vi "Data Filter.vi"(9 "ZeroOffset":i32, 11 "Data":T1[](array[typedef]) {"Direction" items=["Tx", "Rx"]; "CANType" items=["CAN", "CANFD", "CANFD加速"]}) -> (1 "ZeroOffset out":i32, 3 "Data out":T1[](array[typedef]) {"Direction" items=["Tx", "Rx"]; "CANType" items=["CAN", "CANFD", "CANFD加速"]})   [LabVIEW 2018, in "CAN FD.lvlib"]
uses:
  CAN FD.lvlib
  Typedef/CAN Data.ctl
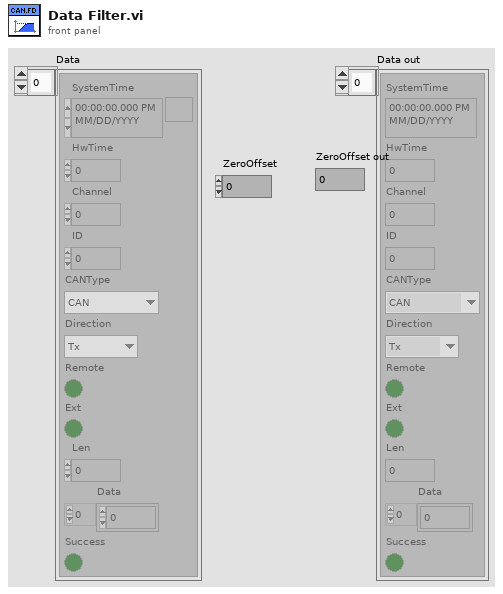
[diagram p1: front panel]
types:
  T1 = typedef "CAN FD.lvlib/CAN Data.ctl" = cluster{"SystemTime":timestamp, "HwTime":dbl, "Channel":u8, "ID":u32, "CANType":i16, "Direction":i16, "Remote":bool, "Ext":bool, "Len":u8, "Data":u8[], "Success":bool}
  T2 = cluster{"Channel":u8, "CANType":i16, "ID":u32, "Direction":i16}[]
  T3 = typedef "CAN FD.lvlib/Config.ctl" = cluster{"TimeFormat":u16, "ID Format":u16, "Data Format":u16, "ListLen":u32}
  T4 = typedef "CAN FD.lvlib/ListFilter.ctl" = cluster{"Timestamp":string, "Channel":string, "ID":string, "Type":i16, "Format":i16, "CANType":i16, "Direction":i16, "Len":string, "Data":string}
  T5 = cluster{"Channel":u8, "CANType":i16, "ID":u32, "Direction":i16}
  T6 = cluster{cluster{"Channel":u8, "CANType":i16, "ID":u32, "Direction":i16}, i32}
  T7 = cluster{cluster{"Channel":u8, "CANType":i16, "ID":u32, "Direction":i16}, i32}[]
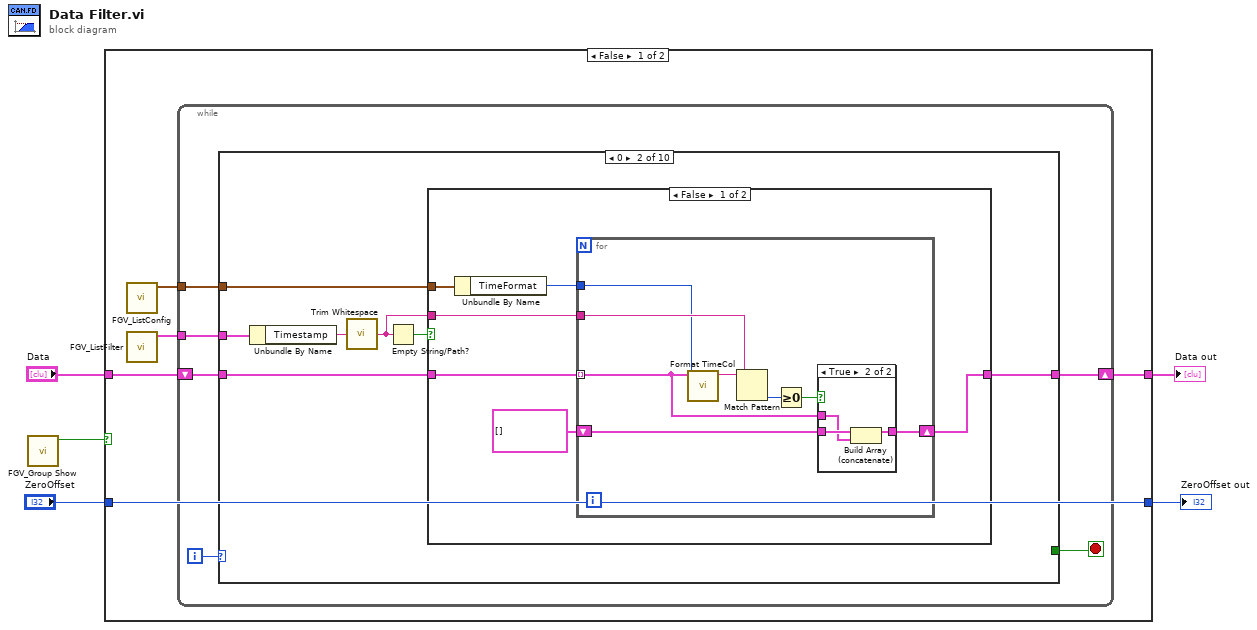
[diagram p0: block diagram]
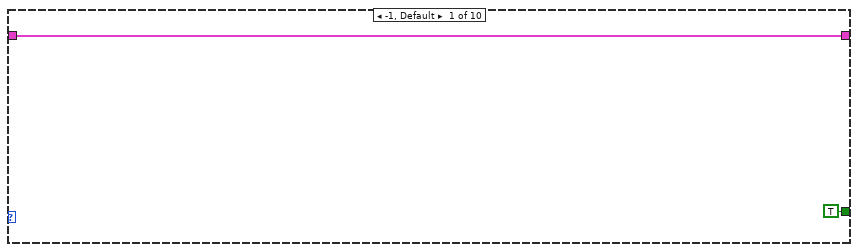
[diagram p2: hidden frame]
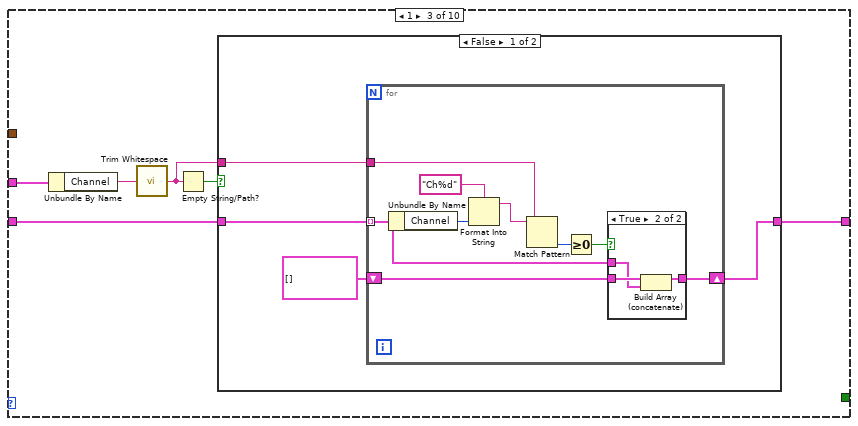
[diagram p5: hidden frame]
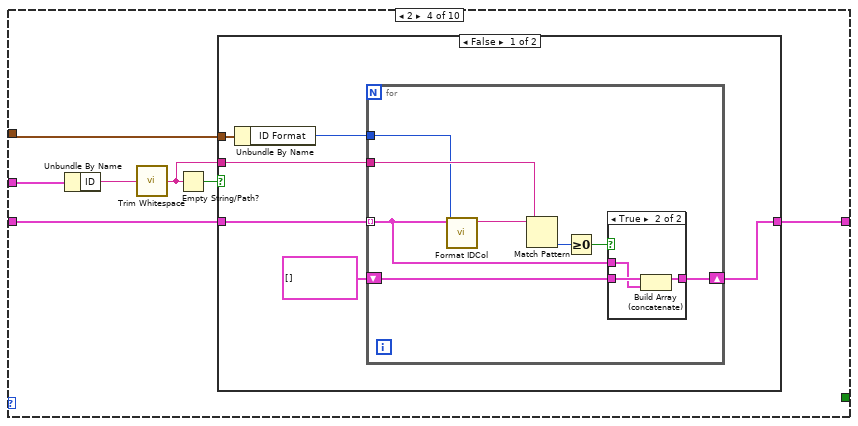
[diagram p8: hidden frame]
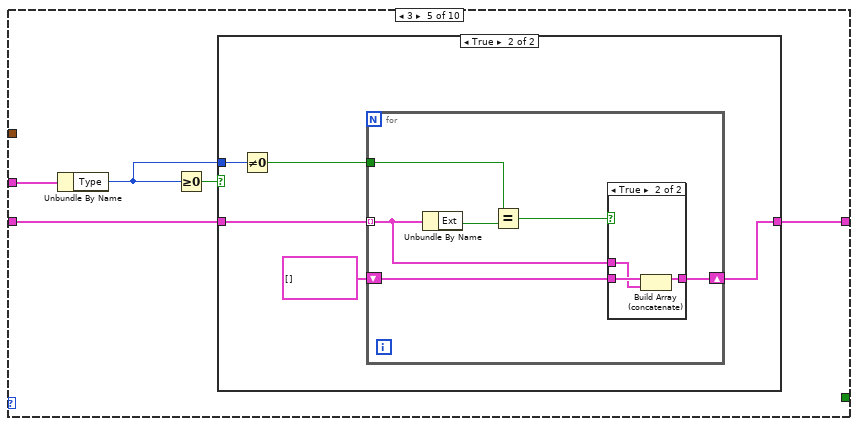
[diagram p11: hidden frame]
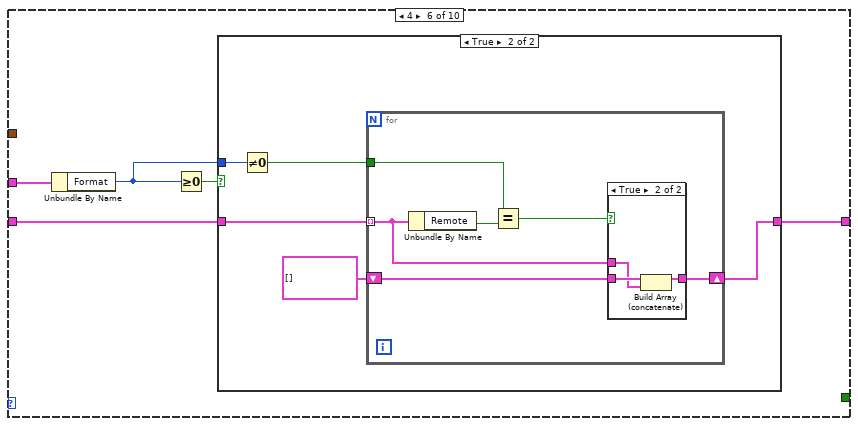
[diagram p14: hidden frame]
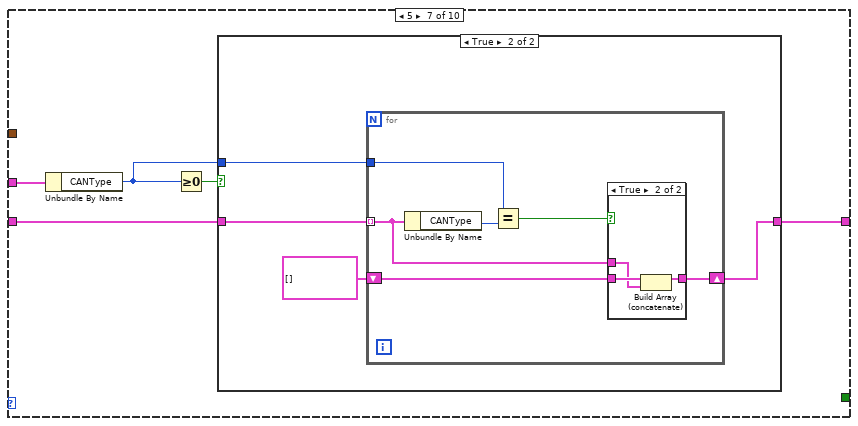
[diagram p17: hidden frame]
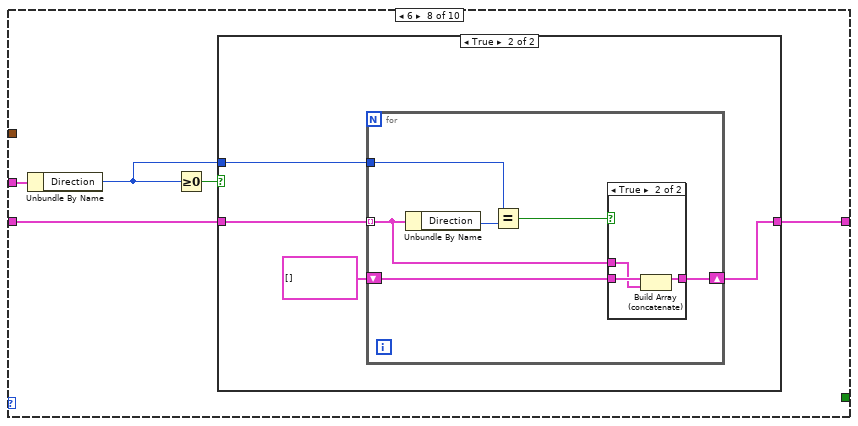
[diagram p20: hidden frame]
diagram:
  n1 = call "FGV_Group Show.vi"() -> ("Group Show"=w4:bool)  [unwired: 10 in, 1 out]
  n2 = case shown="False" w4 {
    tunnel: "Data" -> [w10 w236]
    tunnel: [w9 w228] -> w5
    tunnel: "ZeroOffset" -> [w6 _]
    tunnel: [w6 _] -> w2
    frame False {
      n3 = call "FGV_ListConfig.vi"() -> ("Config out"=w7:T3)  [unwired: 10 in, 1 out]
      n4 = call "FGV_ListFilter.vi"() -> ("Filter out"=w8:T4)  [unwired: 10 in, 1 out]
      n5 = while {
        shift-right: [w14] -> w9
        shift-left: w10 -> [w13]
        tunnel: w8 -> [w12]
        tunnel: w7 -> [w11]
        i -> [w16]
        stop <- w15 stop-if-true
        n6 = case shown="0" w16 {
          tunnel: [TRUE _ _ _ _ _ _ _ _ _] -> w15
          tunnel: [w17 w22 w47 w72 w98 w119 w140 w161 w179 w204] -> w14
          tunnel: w13 -> [w17 w21 w46 w71 w97 w118 w139 w160 w178 w203]
          tunnel: w12 -> [_ w25 w50 w75 w99 w120 w141 w158 w182 w207]
          tunnel: w11 -> [_ w19 _ w69 _ _ _ _ _ w201]
          frame -1, Default {
          }
          frame 0 {
            n7 = Unbundle By Name(w25) -> ("Timestamp"=w24:string)
            n8 = call <vilib>:"Trim Whitespace.vi"("string"=w24) -> ("trimmed string"=w20:string)  [unwired: 1 in]
            n9 = Empty String/Path?(string/path=w20) -> (empty?=w23:bool)
            n10 = case shown="False" w23 {
              tunnel: [w28 w44] -> w22
              tunnel: w21 -> [w31 w44]
              tunnel: w20 -> [w30 _]
              tunnel: w19 -> [w27 _]
              frame False {
                n11 = Unbundle By Name(w27) -> ("TimeFormat"=w26:u16)
                n12 = for {
                  tunnel: w31 -> [w34] mode=indexing
                  tunnel: w30 -> [w38]
                  shift-right: [w33] -> w28
                  shift-left: T1[] [] ("Data") -> [w35]
                  tunnel: w26 -> [w32]
                  n13 = call "Format TimeCol.vi"("TimeFormat"=w32, "Data"=w34) -> ("Time str"=w39:string)  [unwired: 9 in]
                  n14 = Match Pattern(string=w39, regular expression=w38) -> (offset past match=w37:i32)  [unwired: 1 in, 3 out]
                  n15 = Greater Or Equal To 0?(x=w37) -> (x >= 0?=w36:bool)
                  n16 = case shown="True" w36 {
                    tunnel: w35 -> [w40 w43]
                    tunnel: w34 -> [_ w42]
                    tunnel: [w40 w41] -> w33
                    frame False {
                    }
                    frame True {
                      n17 = Build Array (concatenate)(w43, w42) -> (w41:T1[])
                    }
                  }
                }
              }
              frame True {
              }
            }
          }
          frame 1 {
            n18 = Unbundle By Name(w50) -> ("Channel"=w49:string)
            n19 = call <vilib>:"Trim Whitespace.vi"("string"=w49) -> ("trimmed string"=w45:string)  [unwired: 1 in]
            n20 = Empty String/Path?(string/path=w45) -> (empty?=w48:bool)
            n21 = case shown="False" w48 {
              tunnel: [w51 w68] -> w47
              tunnel: w46 -> [w54 w68]
              tunnel: w45 -> [w53 _]
              frame False {
                n22 = for {
                  tunnel: w54 -> [w58] mode=indexing
                  tunnel: w53 -> [w63]
                  shift-right: [w59] -> w51
                  shift-left: T1[] [] ("Data") -> [w60]
                  n23 = Unbundle By Name(w58) -> ("Channel"=w57:u8)
                  n24 = Format Into String(format string="Ch%d" ("格式字符串"), w57) -> (resulting string=w55:string)  [unwired: 2 in, 1 out]
                  n25 = Match Pattern(string=w55, regular expression=w63) -> (offset past match=w62:i32)  [unwired: 1 in, 3 out]
                  n26 = Greater Or Equal To 0?(x=w62) -> (x >= 0?=w61:bool)
                  n27 = case shown="True" w61 {
                    tunnel: w60 -> [w64 w67]
                    tunnel: w58 -> [_ w66]
                    tunnel: [w64 w65] -> w59
                    frame False {
                    }
                    frame True {
                      n28 = Build Array (concatenate)(w67, w66) -> (w65:T1[])
                    }
                  }
                }
              }
              frame True {
              }
            }
          }
          frame 2 {
            n29 = Unbundle By Name(w75) -> ("ID"=w74:string)
            n30 = call <vilib>:"Trim Whitespace.vi"("string"=w74) -> ("trimmed string"=w70:string)  [unwired: 1 in]
            n31 = Empty String/Path?(string/path=w70) -> (empty?=w73:bool)
            n32 = case shown="False" w73 {
              tunnel: [w78 w94] -> w72
              tunnel: w71 -> [w81 w94]
              tunnel: w70 -> [w80 _]
              tunnel: w69 -> [w77 _]
              frame False {
                n33 = Unbundle By Name(w77) -> ("ID Format"=w76:u16)
                n34 = for {
                  tunnel: w81 -> [w84] mode=indexing
                  tunnel: w80 -> [w89]
                  shift-right: [w85] -> w78
                  shift-left: T1[] [] ("Data") -> [w86]
                  tunnel: w76 -> [w83]
                  n35 = call "Format IDCol.vi"("ID Format"=w83, "Data"=w84) -> ("ID str"=w82:string)  [unwired: 9 in]
                  n36 = Match Pattern(string=w82, regular expression=w89) -> (offset past match=w88:i32)  [unwired: 1 in, 3 out]
                  n37 = Greater Or Equal To 0?(x=w88) -> (x >= 0?=w87:bool)
                  n38 = case shown="True" w87 {
                    tunnel: w86 -> [w90 w93]
                    tunnel: w84 -> [_ w92]
                    tunnel: [w90 w91] -> w85
                    frame False {
                    }
                    frame True {
                      n39 = Build Array (concatenate)(w93, w92) -> (w91:T1[])
                    }
                  }
                }
              }
              frame True {
              }
            }
          }
          frame 3 {
            n40 = Unbundle By Name(w99) -> ("Type"=w95:i16)
            n41 = Greater Or Equal To 0?(x=w95) -> (x >= 0?=w96:bool)
            n42 = case shown="True" w96 {
              tunnel: [w100 w103] -> w98
              tunnel: w97 -> [w100 w105]
              tunnel: w95 -> [_ w102]
              frame False {
              }
              frame True {
                n43 = Not Equal To 0?(x=w102) -> (x != 0?=w101:bool)
                n44 = for {
                  tunnel: w105 -> [w109] mode=indexing
                  shift-right: [w110] -> w103
                  shift-left: T1[] [] ("Data") -> [w111]
                  tunnel: w101 -> [w107]
                  n45 = Unbundle By Name(w109) -> ("Ext"=w108:bool)
                  n46 = Equal?(x=w107, y=w108) -> (x = y?=w106:bool)
                  n47 = case shown="True" w106 {
                    tunnel: w111 -> [w112 w115]
                    tunnel: w109 -> [_ w114]
                    tunnel: [w112 w113] -> w110
                    frame False {
                    }
                    frame True {
                      n48 = Build Array (concatenate)(w115, w114) -> (w113:T1[])
                    }
                  }
                }
              }
            }
          }
          frame 4 {
            n49 = Unbundle By Name(w120) -> ("Format"=w116:i16)
            n50 = Greater Or Equal To 0?(x=w116) -> (x >= 0?=w117:bool)
            n51 = case shown="True" w117 {
              tunnel: [w121 w124] -> w119
              tunnel: w118 -> [w121 w126]
              tunnel: w116 -> [_ w123]
              frame False {
              }
              frame True {
                n52 = Not Equal To 0?(x=w123) -> (x != 0?=w122:bool)
                n53 = for {
                  tunnel: w126 -> [w130] mode=indexing
                  shift-right: [w131] -> w124
                  shift-left: T1[] [] ("Data") -> [w132]
                  tunnel: w122 -> [w128]
                  n54 = Unbundle By Name(w130) -> ("Remote"=w129:bool)
                  n55 = Equal?(x=w128, y=w129) -> (x = y?=w127:bool)
                  n56 = case shown="True" w127 {
                    tunnel: w132 -> [w133 w136]
                    tunnel: w130 -> [_ w135]
                    tunnel: [w133 w134] -> w131
                    frame False {
                    }
                    frame True {
                      n57 = Build Array (concatenate)(w136, w135) -> (w134:T1[])
                    }
                  }
                }
              }
            }
          }
          frame 5 {
            n58 = Unbundle By Name(w141) -> ("CANType"=w137:i16)
            n59 = Greater Or Equal To 0?(x=w137) -> (x >= 0?=w138:bool)
            n60 = case shown="True" w138 {
              tunnel: [w142 w144] -> w140
              tunnel: w139 -> [w142 w146]
              tunnel: w137 -> [_ w143]
              frame False {
              }
              frame True {
                n61 = for {
                  tunnel: w146 -> [w150] mode=indexing
                  shift-right: [w151] -> w144
                  shift-left: T1[] [] ("Data") -> [w152]
                  tunnel: w143 -> [w148]
                  n62 = Unbundle By Name(w150) -> ("CANType"=w149:i16)
                  n63 = Equal?(x=w148, y=w149) -> (x = y?=w147:bool)
                  n64 = case shown="True" w147 {
                    tunnel: w152 -> [w153 w156]
                    tunnel: w150 -> [_ w155]
                    tunnel: [w153 w154] -> w151
                    frame False {
                    }
                    frame True {
                      n65 = Build Array (concatenate)(w156, w155) -> (w154:T1[])
                    }
                  }
                }
              }
            }
          }
          frame 6 {
            n66 = Unbundle By Name(w158) -> ("Direction"=w157:i16)
            n67 = Greater Or Equal To 0?(x=w157) -> (x >= 0?=w159:bool)
            n68 = case shown="True" w159 {
              tunnel: [w162 w164] -> w161
              tunnel: w160 -> [w162 w166]
              tunnel: w157 -> [_ w163]
              frame False {
              }
              frame True {
                n69 = for {
                  tunnel: w166 -> [w170] mode=indexing
                  shift-right: [w171] -> w164
                  shift-left: T1[] [] ("Data") -> [w172]
                  tunnel: w163 -> [w168]
                  n70 = Unbundle By Name(w170) -> ("Direction"=w169:i16)
                  n71 = Equal?(x=w168, y=w169) -> (x = y?=w167:bool)
                  n72 = case shown="True" w167 {
                    tunnel: w172 -> [w173 w176]
                    tunnel: w170 -> [_ w175]
                    tunnel: [w173 w174] -> w171
                    frame False {
                    }
                    frame True {
                      n73 = Build Array (concatenate)(w176, w175) -> (w174:T1[])
                    }
                  }
                }
              }
            }
          }
          frame 7 {
            n74 = Unbundle By Name(w182) -> ("Len"=w181:string)
            n75 = call <vilib>:"Trim Whitespace.vi"("string"=w181) -> ("trimmed string"=w177:string)  [unwired: 1 in]
            n76 = Empty String/Path?(string/path=w177) -> (empty?=w180:bool)
            n77 = case shown="False" w180 {
              tunnel: [w183 w200] -> w179
              tunnel: w178 -> [w186 w200]
              tunnel: w177 -> [w185 _]
              frame False {
                n78 = for {
                  tunnel: w186 -> [w190] mode=indexing
                  tunnel: w185 -> [w195]
                  shift-right: [w191] -> w183
                  shift-left: T1[] [] ("Data") -> [w192]
                  n79 = Unbundle By Name(w190) -> ("Len"=w189:u8)
                  n80 = Format Into String(format string="%d" ("格式字符串"), w189) -> (resulting string=w187:string)  [unwired: 2 in, 1 out]
                  n81 = Match Pattern(string=w187, regular expression=w195) -> (offset past match=w194:i32)  [unwired: 1 in, 3 out]
                  n82 = Greater Or Equal To 0?(x=w194) -> (x >= 0?=w193:bool)
                  n83 = case shown="True" w193 {
                    tunnel: w192 -> [w196 w199]
                    tunnel: w190 -> [_ w198]
                    tunnel: [w196 w197] -> w191
                    frame False {
                    }
                    frame True {
                      n84 = Build Array (concatenate)(w199, w198) -> (w197:T1[])
                    }
                  }
                }
              }
              frame True {
              }
            }
          }
          frame 8 {
            n85 = Unbundle By Name(w207) -> ("Data"=w206:string)
            n86 = call <vilib>:"Trim Whitespace.vi"("string"=w206) -> ("trimmed string"=w202:string)  [unwired: 1 in]
            n87 = Empty String/Path?(string/path=w202) -> (empty?=w205:bool)
            n88 = case shown="False" w205 {
              tunnel: [w210 w226] -> w204
              tunnel: w203 -> [w213 w226]
              tunnel: w202 -> [w212 _]
              tunnel: w201 -> [w209 _]
              frame False {
                n89 = Unbundle By Name(w209) -> ("Data Format"=w208:u16)
                n90 = for {
                  tunnel: w213 -> [w216] mode=indexing
                  tunnel: w212 -> [w221]
                  shift-right: [w217] -> w210
                  shift-left: T1[] [] ("Data") -> [w218]
                  tunnel: w208 -> [w214]
                  n91 = call "Format DataCol.vi"("Data Format"=w214, "Data"=w216) -> ("ID str"=w215:string)  [unwired: 9 in]
                  n92 = Match Pattern(string=w215, regular expression=w221) -> (offset past match=w220:i32)  [unwired: 1 in, 3 out]
                  n93 = Greater Or Equal To 0?(x=w220) -> (x >= 0?=w219:bool)
                  n94 = case shown="True" w219 {
                    tunnel: w218 -> [w222 w225]
                    tunnel: w216 -> [_ w224]
                    tunnel: [w222 w223] -> w217
                    frame False {
                    }
                    frame True {
                      n95 = Build Array (concatenate)(w225, w224) -> (w223:T1[])
                    }
                  }
                }
              }
              frame True {
              }
            }
          }
        }
      }
    }
    frame True {
      n96 = Array Size(array=w236) -> (size(s)=w235:i32)
      n97 = Decrement(x=w235) -> (x-1=w234:i32)
      n98 = for {
        N: w235 -> [_]
        tunnel: w236 -> [w258]
        tunnel: w234 -> [w256]
        shift-right: [w249] -> w232
        shift-left: T2 [] -> [w251]
        shift-right: [w248] -> w229
        shift-left: T1[] [] ("Data") -> [w247]
        i -> [w257]
        n99 = Subtract(x=w256, y=w257) -> (x-y=w255:i32)
        n100 = Index Array(array=w258, index=w255) -> (element=w246:T1)
        n101 = Unbundle By Name(w246) -> ("Channel"=w254:u8, "CANType"=w245:i16, "ID"=w244:u32, "Direction"=w253:i16)
        n102 = Bundle("Channel"=w254, "CANType"=w245, "ID"=w244, "Direction"=w253) -> (w250:T5)  [unwired: 1 in]
        n103 = Search 1D Array(1D array=w251, element=w250) -> (index of element=w252:i32)  [unwired: 1 in]
        n104 = case shown="..-1" w252 {
          tunnel: w251 -> [w260 w266]
          tunnel: w250 -> [_ w265]
          tunnel: [w260 w264] -> w249
          tunnel: [w259 w262] -> w248
          tunnel: w247 -> [w259 w263]
          tunnel: w246 -> [_ w261]
          frame 0, Default {
          }
          frame ..-1 {
            n105 = Build Array (concatenate)(w266, w265) -> (w264:T2)
            n106 = Build Array (concatenate)(w263, w261) -> (w262:T1[])
          }
        }
      }
      n107 = for {
        tunnel: w232 -> [w243] mode=indexing
        tunnel: [w242] -> w231 mode=indexing
        i -> [w241]
        n108 = Bundle(w243, w241) -> (w242:T6)  [unwired: 1 in]
      }
      n109 = Sort 1D Array(array=w231) -> (sorted array=w230:T7)
      n110 = for {
        tunnel: w230 -> [w240] mode=indexing
        tunnel: w229 -> [w239]
        tunnel: [w237] -> w228 mode=indexing
        n111 = Unbundle(w240) -> (w238:i32)  [unwired: 1 out]
        n112 = Index Array(array=w239, index=w238) -> (element=w237:T1)
      }
    }
  }
  "Data out" <- w5
  "ZeroOffset out" <- w2
